vi "Configure Hcopy.vi"() -> ()   [LabVIEW 2018, in "Suita SPAW7000.lvlib"]
uses:
  <instrlib>/Suita SPAW7000/Suita SPAW7000.lvlib
panel:
  in  "option":u16(ring) items=["AUTO", "EXEC"]
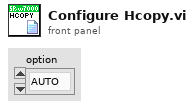
[diagram p1: front panel]
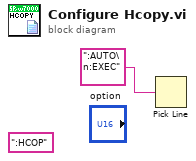
[diagram p0: block diagram]
diagram:
  (unwired) ":HCOP"
  n1 = Pick Line(multi-line string=":AUTO\n:EXEC") -> ()  [unwired: 2 in, 1 out]
